vi "vi.SetVariantName.vi"(0 "Variant in":variant, 7 "Name":string, 11 "error in":errorcluster) -> (4 "Named Variant":variant, 15 "error out":errorcluster)   [LabVIEW 2014, in "GLue.lvlib" / "class.GLue.lvclass"]
uses:
  class.GLue.lvclass
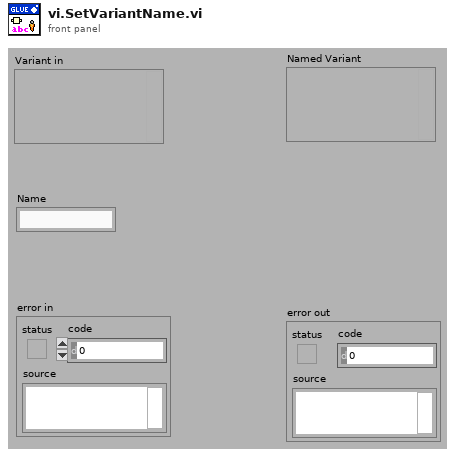
[diagram p1: front panel]
types:
  T1 = cluster{"length":u16, "private":u8, "type":enum8{"<Null>", "I8", "I16", "I32", "I64", "U8", "U16", "U32", "U64", "SGL", "DBL", "EXT", "CSG", "CDB", "CXT", "0x0F", "0x10", "0x11", "0x12", "0x13", "0x14", "Enum U8", "Enum U16", "Enum U32", "Enum U64", "SGL PQ", "DBL PQ", "EXT PQ", "CSG PQ", "CDB PQ", "CXT PQ", "0x1F", "0x20", "Boolean", "0x22", "0x23", "0x24", "0x25", "0x26", "0x27", "0x28", "0x29", "0x2A", "0x2B", "0x2C", "0x2D", "0x2E", "0x2F", "String", "0x31", "Path", "Pict", "0x34", "0x35", "0x36", "DAQ", "0x38", "0x39", "0x3A", "0x3B", "0x3C", "0x3D", "0x3E", "0x3F", "Array", "0x41", "0x42", "0x43", "0x44", "0x45", "0x46", "0x47", "0x48", "0x49", "0x4A", "0x4B", "0x4C", "0x4D", "0x4E", "0x4F", "Cluster", "0x51", "0x52", "Variant", "Waveform", "0x55", "0x56", "0x57", "0x58", "0x59", "0x5A", "0x5B", "0x5C", "0x5D", "0x5E", "0x5F", "0x60", "0x61", "0x62", "0x63", "0x64", "0x65", "0x66", "0x67", "0x68", "0x69", "0x6A", "0x6B", "0x6C", "0x6D", "0x6E", "0x6F", "Refnum"}, "# elements":u16}
  T2 = enum8{"<Null>", "I8", "I16", "I32", "I64", "U8", "U16", "U32", "U64", "SGL", "DBL", "EXT", "CSG", "CDB", "CXT", "0x0F", "0x10", "0x11", "0x12", "0x13", "0x14", "Enum U8", "Enum U16", "Enum U32", "Enum U64", "SGL PQ", "DBL PQ", "EXT PQ", "CSG PQ", "CDB PQ", "CXT PQ", "0x1F", "0x20", "Boolean", "0x22", "0x23", "0x24", "0x25", "0x26", "0x27", "0x28", "0x29", "0x2A", "0x2B", "0x2C", "0x2D", "0x2E", "0x2F", "String", "0x31", "Path", "Pict", "0x34", "0x35", "0x36", "DAQ", "0x38", "0x39", "0x3A", "0x3B", "0x3C", "0x3D", "0x3E", "0x3F", "Array", "0x41", "0x42", "0x43", "0x44", "0x45", "0x46", "0x47", "0x48", "0x49", "0x4A", "0x4B", "0x4C", "0x4D", "0x4E", "0x4F", "Cluster", "0x51", "0x52", "Variant", "Waveform", "0x55", "0x56", "0x57", "0x58", "0x59", "0x5A", "0x5B", "0x5C", "0x5D", "0x5E", "0x5F", "0x60", "0x61", "0x62", "0x63", "0x64", "0x65", "0x66", "0x67", "0x68", "0x69", "0x6A", "0x6B", "0x6C", "0x6D", "0x6E", "0x6F", "Refnum"}
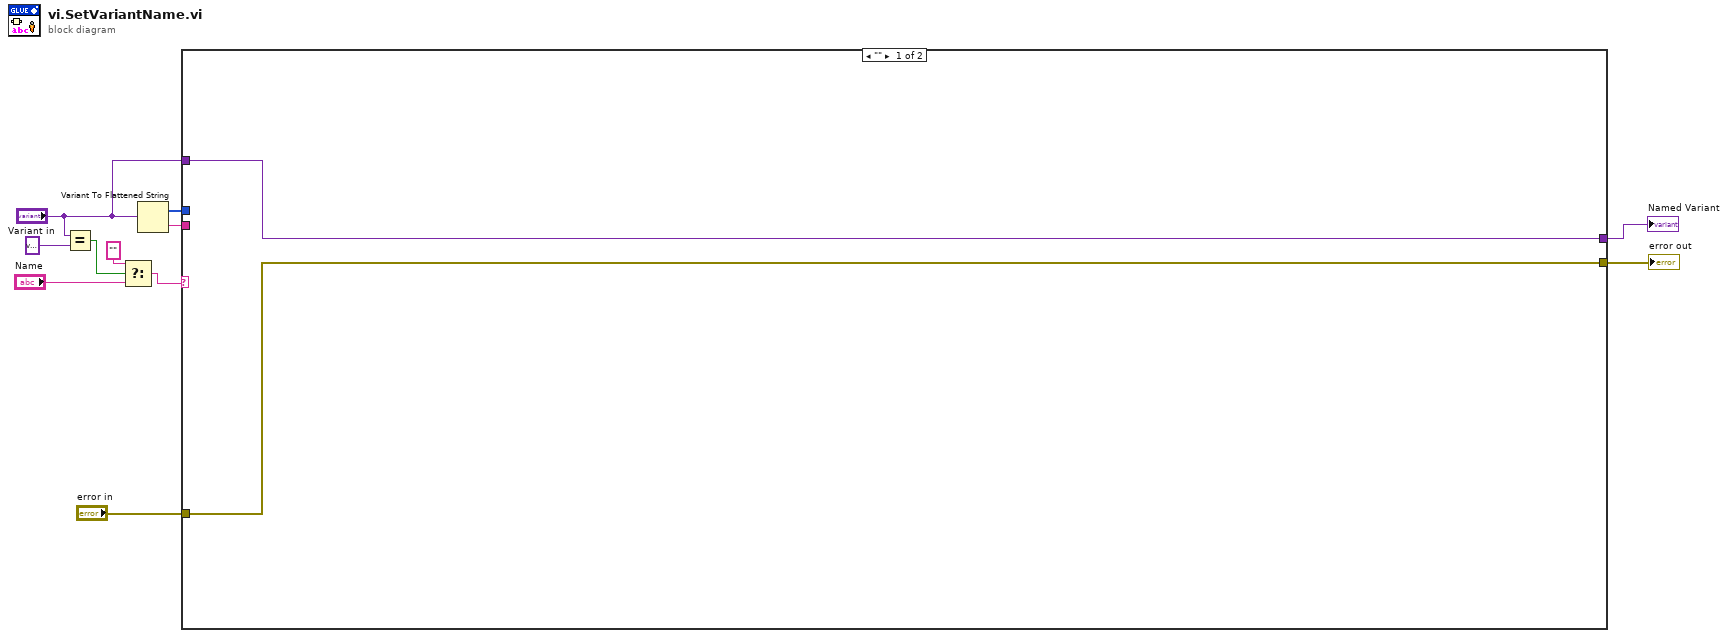
[diagram p0: block diagram]
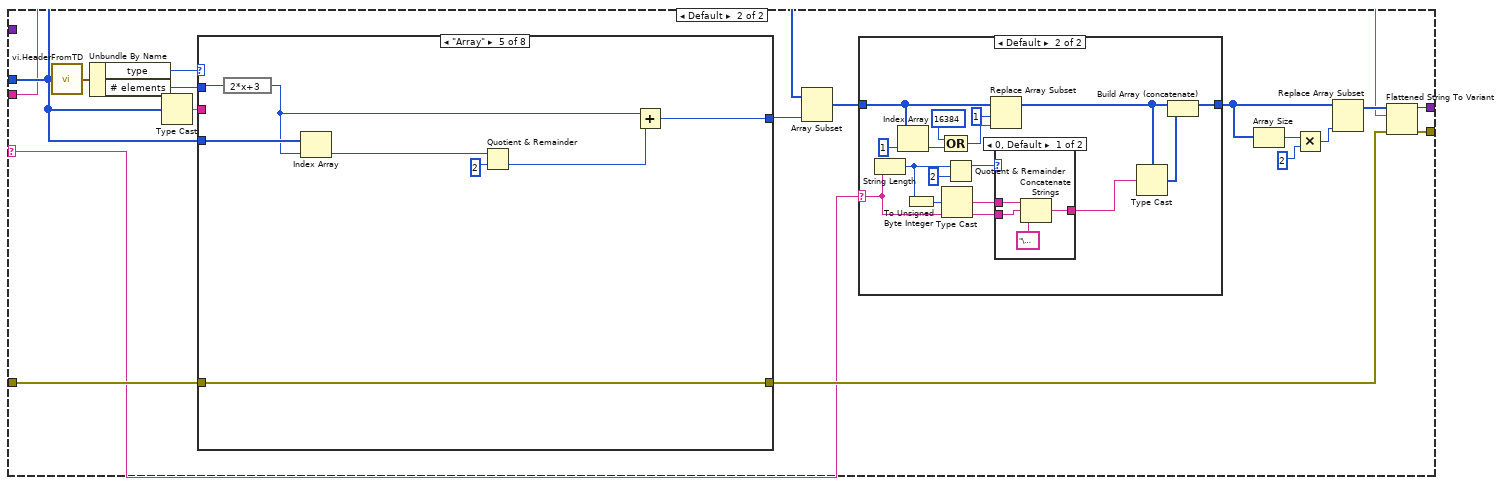
[diagram p2: hidden frame]
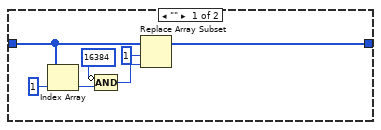
[diagram p3: hidden frame]
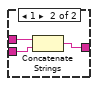
[diagram p4: hidden frame]
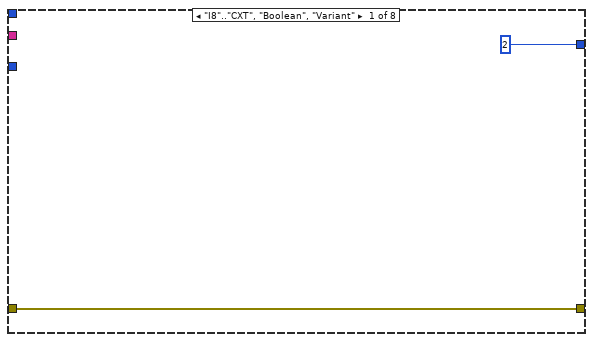
[diagram p5: hidden frame]
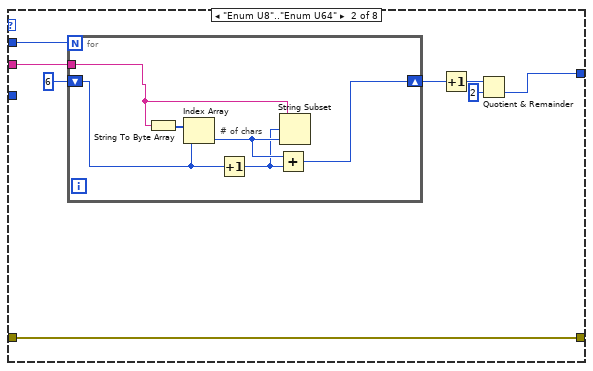
[diagram p6: hidden frame]
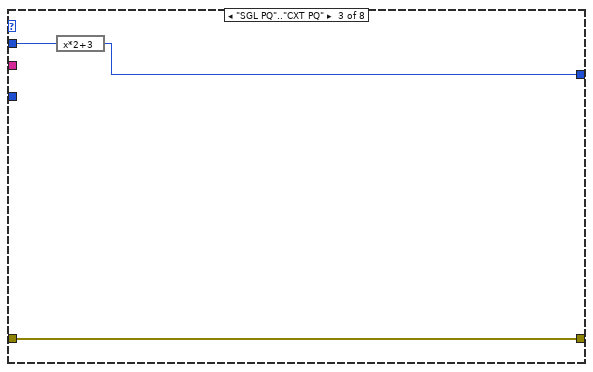
[diagram p7: hidden frame]
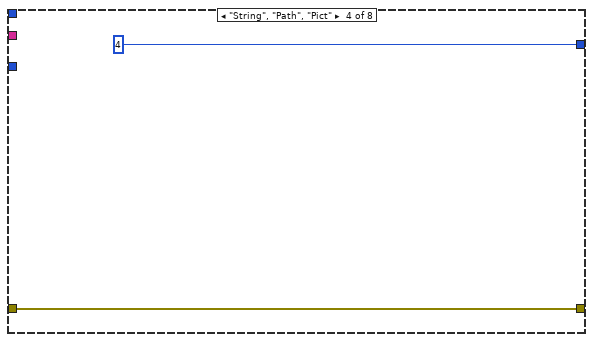
[diagram p8: hidden frame]
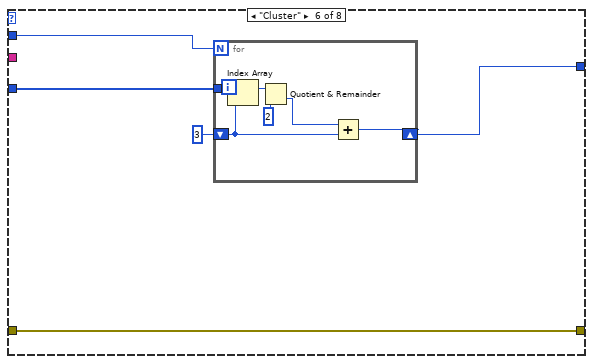
[diagram p9: hidden frame]
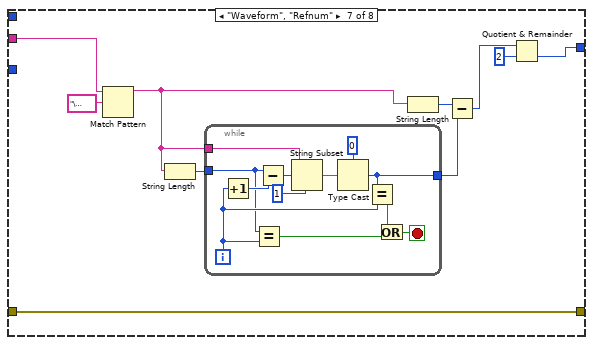
[diagram p10: hidden frame]
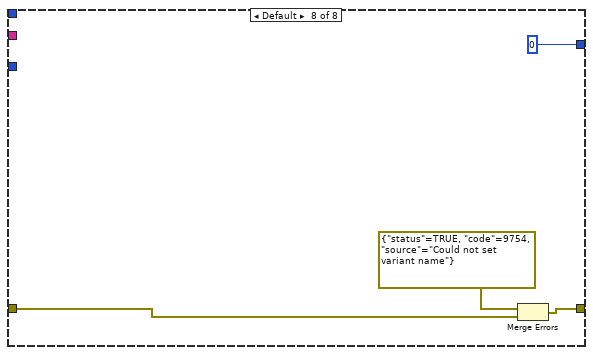
[diagram p11: hidden frame]
diagram:
  n1 = Equal?(x="Variant in", y=variant ("variant")) -> (x = y?=w3:bool)
  n2 = Select(t="" ("Name"), s=w3, f="Name") -> (s? t:f=w1:string)
  n3 = Variant To Flattened String(Variant="Variant in") -> (data string=w7:string, 1:w10:i16[])
  n4 = case shown="\"\"" w1 {
    selector: w1 -> [_ w14]
    tunnel: "error in" -> [w13 w27]
    tunnel: w10 -> [_ w25]
    tunnel: [w13 w17] -> w9
    tunnel: [w12 w16] -> w8
    tunnel: w7 -> [_ w15]
    tunnel: "Variant in" -> [w12 _]
    frame "" {
    }
    frame Default {
      n5 = call "vi.HeaderFromTD.vi"("Type Descriptor"=w25) -> ("Type Descriptor Header"=w31:T1)  [unwired: 4 in]
      n6 = Unbundle By Name(w31) -> ("type"=w30:T2, "# elements"=w29:u16)
      n7 = Type Cast(x=w25) -> (*(type *) &x=w28:string)  [unwired: 1 in]
      n8 = case shown="\"Array\"" w30 {
        tunnel: [w62 w65 w78 w81 w83 w91 w109 w125] -> w18
        tunnel: w28 -> [_ w64 _ _ _ _ w103 _]
        tunnel: w29 -> [_ w69 w80 _ w90 w95 _ _]
        tunnel: w25 -> [_ _ _ _ w89 w94 _ _]
        tunnel: [2 ("offset (0)") w66 w79 4 ("offset (0)") w84 w92 w110 0 ("PString Offset")] -> w26
        tunnel: w27 -> [w62 w65 w78 w81 w83 w91 w109 w126]
        frame "I8".."CXT", "Boolean", "Variant" {
        }
        frame "Enum U8".."Enum U64" {
          n9 = for {
            N: w69 -> [_]
            tunnel: w64 -> [w74]
            shift-right: [w72] -> w70
            shift-left: 6 -> [w73]
            # "# of chars"
            n10 = String To Byte Array(string=w74) -> (unsigned byte array=w75:u8[])
            n11 = Index Array(array=w75, index=w73) -> (element=w77:u8)
            n12 = Increment(x=w73) -> (x+1=w76:i32)
            n13 = Add(x=w77, y=w76) -> (x+y=w72:i32)
            n14 = String Subset(string=w74, offset (0)=w76, length (rest)=w77) -> ()  [unwired: 1 out]
          }
          n15 = Increment(x=w70) -> (x+1=w67:i32)
          n16 = Quotient & Remainder(x=w67, y=2) -> (floor(x/y)=w66:i32)  [unwired: 1 out]
        }
        frame "SGL PQ".."CXT PQ" {
          n17 = expression code="x*2+3"(w80) -> (w79:u16)
        }
        frame "String", "Path", "Pict" {
        }
        frame "Array" {
          n18 = expression code="2*x+3"(w90) -> (w85:u16)
          n19 = Index Array(array=w89, index=w85) -> (element=w87:i16)
          n20 = Quotient & Remainder(x=w87, y=u16 2) -> (floor(x/y)=w86:u16)  [unwired: 1 out]
          n21 = Add(x=w85, y=w86) -> (x+y=w84:u16)
        }
        frame "Cluster" {
          n22 = for {
            N: w95 -> [_]
            shift-right: [w100] -> w92
            shift-left: i16 3 -> [w99]
            tunnel: w94 -> [w101]
            n23 = Index Array(array=w101, index=w99) -> (element=w97:i16)
            n24 = Quotient & Remainder(x=w97, y=i16 2) -> (floor(x/y)=w98:i16)  [unwired: 1 out]
            n25 = Add(x=w98, y=w99) -> (x+y=w100:i16)
          }
        }
        frame "Waveform", "Refnum" {
          n26 = Match Pattern(string=w103, regular expression="\u0000$" ("*(type *) &x")) -> (before substring=w105:string)  [unwired: 1 in, 3 out]
          n27 = String Length(string=w105) -> (length=w104:i32)
          n28 = while {
            tunnel: [w118] -> w108
            tunnel: w104 -> [w113]
            tunnel: w105 -> [w122]
            i -> [w116]
            stop <- w115 stop-if-true
            n29 = Increment(x=w116) -> (x+1=w117:i32)
            n30 = Equal?(x=w113, y=w116) -> (x = y?=w112:bool)
            n31 = Subtract(x=w113, y=w117) -> (x-y=w121:i32)
            n32 = String Subset(string=w122, offset (0)=w121, length (rest)=1 ("length (rest)")) -> (substring=w120:string)
            n33 = Type Cast(type=u8 0, x=w120) -> (*(type *) &x=w118:u8)
            n34 = Equal?(x=w118, y=w116) -> (x = y?=w114:bool)
            n35 = Or(x=w114, y=w112) -> (x .or. y?=w115:bool)
          }
          n36 = String Length(string=w105) -> (length=w107:i32)
          n37 = Subtract(x=w107, y=w108) -> (x-y=w102:i32)
          n38 = Quotient & Remainder(x=w102, y=2) -> (floor(x/y)=w110:i32)  [unwired: 1 out]
        }
        frame Default {
          n39 = Merge Errors(errorcluster {"status"=TRUE, "code"=9754, "source"="Could not set variant name"} ("error in"), w126) -> (w125:errorcluster)
        }
      }
      n40 = Array Subset(array=w25, length=w26) -> (w24:i16[])  [unwired: 1 in]
      n41 = case shown="Default" w14 {
        selector: w14 -> [_ w46]
        tunnel: w24 -> [w38 w54]
        tunnel: [w33 w43] -> w20
        frame "" {
          n42 = Index Array(array=w38, index=1 ("Index")) -> (element=w36:i16)
          n43 = Compound Arithmetic op=AND(invert i16 16384 ("Input"), w36) -> (w35:i16)
          n44 = Replace Array Subset(array=w38, new element=w35, index=1 ("Index")) -> (w33:i16[])
        }
        frame Default {
          n45 = String Length(string=w46) -> (length=w42:i32)
          n46 = Index Array(array=w54, index=1 ("Index")) -> (element=w50:i16)
          n47 = To Unsigned Byte Integer(number=w42) -> (unsigned 8bit integer=w41:u8)
          n48 = Type Cast(x=w41) -> (*(type *) &x=w40:string)  [unwired: 1 in]
          n49 = Compound Arithmetic op=OR(i16 16384 ("Input"), w50) -> (w52:i16)
          n50 = Quotient & Remainder(x=w42, y=2) -> (x-y*floor(x/y)=w48:i32)  [unwired: 1 out]
          n51 = Replace Array Subset(array=w54, new element=w52, index=1 ("Index")) -> (w44:i16[])
          n52 = case shown="0, Default" w48 {
            tunnel: [w58 w59] -> w47
            tunnel: w46 -> [w57 w60]
            tunnel: w40 -> [w55 w61]
            frame 0, Default {
              n53 = Concatenate Strings(w55, w57, "\u0000" ("Substring")) -> (w58:string)
            }
            frame 1 {
              n54 = Concatenate Strings(w61, w60) -> (w59:string)
            }
          }
          n55 = Type Cast(type=w44, x=w47) -> (*(type *) &x=w45:i16[])
          n56 = Build Array (concatenate)(w44, w45) -> (w43:i16[])
        }
      }
      n57 = Array Size(array=w20) -> (size(s)=w21:i32)
      n58 = Multiply(x=w21, y=2) -> (x*y=w23:i32)
      n59 = Replace Array Subset(array=w20, new element=w23) -> (w19:i16[])  [unwired: 1 in]
      n60 = Flattened String To Variant(4:w18, 6:w15, 7:w19) -> (0:w17:errorcluster, 3:w16:variant)
    }
  }
  "error out" <- w9
  "Named Variant" <- w8
